vi "scale_map.vi"(3 "error in":errorcluster, 4 "Map.DrawArea":T1, 5 "location y":dbl, 6 "location x":dbl) -> (0 "error out":errorcluster, 2 "point(x,y)":cluster{"x":i16, "y":i16})   [LabVIEW 2019, in "Lib_Simx.lvlib"]
doc: "Use to fit the map into the drawing space."
uses:
  Lib_Simx.lvlib
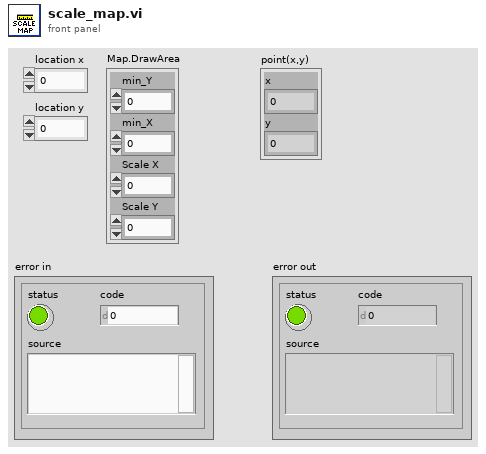
[diagram p1: front panel]
types:
  T1 = cluster{"min_Y":dbl, "min_X":dbl, "Scale X":dbl, "Scale Y":dbl}
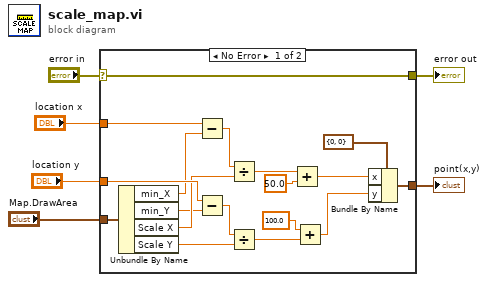
[diagram p0: block diagram]
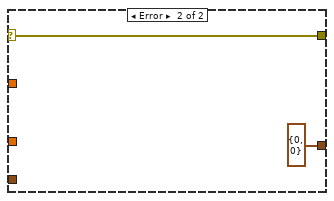
[diagram p2: hidden frame]
diagram:
  n1 = case shown="No Error" "error in" {
    selector: "error in" -> [w17 w26]
    tunnel: [w20 cluster{"x":i16, "y":i16} {"x"=0, "y"=0} ("point(x,y)")] -> w6
    tunnel: "location y" -> [w19 _]
    tunnel: "location x" -> [w18 _]
    tunnel: [w17 w26] -> w2
    tunnel: "Map.DrawArea" -> [w16 _]
    frame No Error {
      n2 = Unbundle By Name(w16) -> ("min_X"=w15:dbl, "min_Y"=w11:dbl, "Scale X"=w14:dbl, "Scale Y"=w13:dbl)
      n3 = Subtract(x=w18, y=w15) -> (x-y=w23:dbl)
      n4 = Subtract(x=w19, y=w11) -> (x-y=w22:dbl)
      n5 = Divide(x=w23, y=w14) -> (x/y=w24:dbl)
      n6 = Divide(x=w22, y=w13) -> (x/y=w12:dbl)
      n7 = Add(x=w24, y=50.0) -> (x+y=w9:dbl)
      n8 = Add(x=100.0, y=w12) -> (x+y=w10:dbl)
      n9 = Bundle By Name(cluster=cluster{"x":i16, "y":i16} {"x"=0, "y"=0} ("point(x,y)"), "x"=w9, "y"=w10) -> (w20:cluster{"x":i16, "y":i16})
    }
    frame Error {
    }
  }
  "point(x,y)" <- w6
  "error out" <- w2
